vi "Send Request.vi"(4 "bank":u8 format="%.0x", 5 "nodeAddr":u16 format="%.0x", 6 "module":u8 format="%.0x", 7 "cmd":T1 items=["NONE", "ROR", "ROL", "MST", "MVP", "SAP", "GAP", "STAP", "RSAP", "SGP", "GGP"], 8 "error in (no error)":errorcluster, 9 "value":u32, 10 "type":u8 format="%.0x", 11 "masterHdl in":T2) -> (0 "error out":errorcluster, 3 "master ref out":T2)   [LabVIEW 2017, in "NI_Robotics_KUKA youBot Host.lvlib"]
uses:
  <vilib>/robotics/KUKA youBot/NI_Robotics_KUKA youBot Host.lvlib
  <vilib>/robotics/KUKA youBot/EtherCAT/LowLevel/Mater Handler.ctl
  <vilib>/robotics/KUKA youBot/EtherCAT/CmdCtrls/Param Cmd.ctl
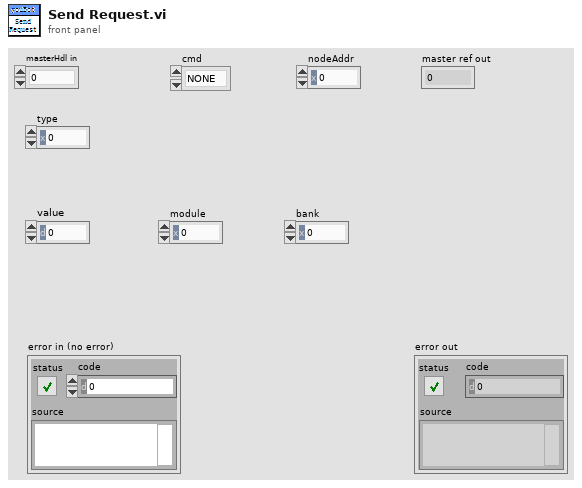
[diagram p1: front panel]
types:
  T1 = typedef "NI_Robotics_KUKA youBot Host.lvlib/Param Cmd.ctl" = u8
  T2 = typedef "NI_Robotics_KUKA youBot Host.lvlib/Mater Handler.ctl" = i32
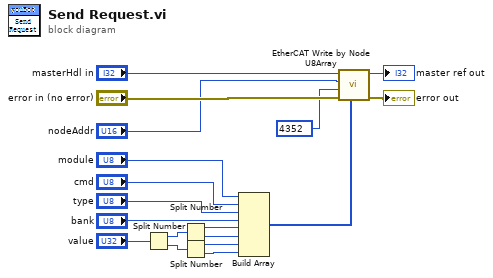
[diagram p0: block diagram]
diagram:
  n1 = Split Number(x="value") -> (hi(x)=w17:u16, lo(x)=w18:u16)
  n2 = Split Number(x=w17) -> (hi(x)=w13:u8, lo(x)=w12:u8)
  n3 = Split Number(x=w18) -> (hi(x)=w11:u8, lo(x)=w10:u8)
  n4 = Build Array("module", "cmd", "type", "bank", w13, w12, w11, w10) -> (w1:T1[])
  n5 = call <vilib>:"EtherCAT Write by Node U8Array.vi"("data"=w1, "error in (no error)"="error in (no error)", "startAddr"=u16 4352 ("nodeAddr"), "nodeAddr"="nodeAddr", "masterHdl in"="masterHdl in") -> ("error out"=→"error out":errorcluster, "masterHdl out"=→"master ref out":T2)  [unwired: 5 in]
